vi "GetTestElement.vi"(8 "Error Out":errorcluster, 10 "Test Index (0)":i32, 11 "Bus Reference":refnum<class "Bus.lvclass">) -> (0 "Error Out":errorcluster, 3 "TestClass":refnum<class "Test.lvclass">)   [LabVIEW 2018]
doc: "This VI gets the specific test element specified by the Test Index."
uses:
  NistPluggableModules/BusClass/Bus.lvclass
  NistPluggableModules/TestClass/Test.lvclass
  NistPluggableModules/BusClass/Bus.lvclass/Bus.ctl
  NistPluggableModules/BusClass/Accessors/Read Test.vi
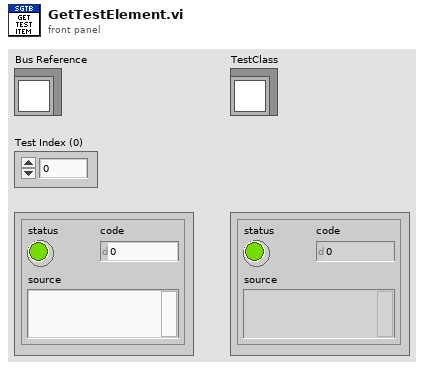
[diagram p1: front panel]
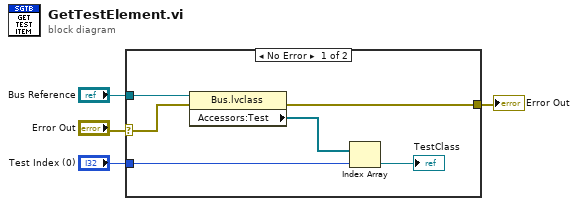
[diagram p0: block diagram]
diagram:
  n1 = case shown="No Error" "Error Out" {
    selector: "Error Out" -> [w9 w11]
    tunnel: [w6 w11] -> w3
    tunnel: "Test Index (0)" -> [w8 _]
    tunnel: "Bus Reference" -> [w7 _]
    frame No Error {
      n2 = property class="Bus.lvclass"(reference=w7, error in=w9) -> (error out=w6:errorcluster, "Accessors:Test"=w10:refnum<class "Test.lvclass">[])  [unwired: 1 out]
      n3 = Index Array(array=w10, index=w8) -> (element=→"TestClass":refnum<class "Test.lvclass">)
    }
    frame Error {
    }
  }
  "Error Out" <- w3
